vi "SerialReadandWrite.vi"() -> ()   [LabVIEW 2018]
doc: "This example performs writes and reads on a serial port, as directed by the user. You can press the Write and Read buttons, and change the Read Count, while the example is running.\n\nThe parameters set for the serial port must match the parameters of the connected instrument or device. In this example, the Read Count parameter specifies the number of bytes that the serial port reads. If there were more bytes at the port than the specified number, those bytes would not be read. If there were less bytes at the port than the specified number, you would receive a timeout error.\n\nThis example expands upon the flow control options for XON and XOFF, allowing the user to choose those control characters. Also, the user can enable or disable a termination character. Some devices require a termination character in order to identify the end of command strings. Some devices send a termination character to signify the end of data to be read. This example shows how you can end the Read operation once a termination character is detected in the buffer and/or append a termination character at the end of the Write data."
uses:
  Program Files (x86)/National Instruments/LabVIEW 2018/examples/Instrument IO/Serial/support/Serial - Settings.ctl
  <vilib>/Instr/_visa.llb/VISA Configure Serial Port (Instr).vi
panel:
  out "unsigned byte array":u8[](array[numeric])
  in  "VISA resource name":refnum<visa-resource-name>="COM1"
  in  "Serial Settings":T1={"baud rate"=9600, "data bits"=8, "parity"=enum."None", "stop bits"=10, "flow control"=0} {"flow control" items=["None"=0, "XON/XOFF"=1, "RTS/CTS"=2, "DTR/DSR"=4]; "stop bits" items=["1.0"=10, "1.5"=15, "2.0"=20]; "data bits" min=5 max=8 step=1; "baud rate" items=["75"=75, "110"=110, "134"=134, "150"=150, "300"=300, "600"=600, "1200"=1200, "1800"=1800, "2400"=2400, "4800"=4800, "7200"=7200, "9600"=9600, "14400"=14400, "19200"=19200, "28800"=28800, "38400"=38400, "56000"=56000, "57600"=57600, "115200"=115200, "128000"=128000, "230400"=230400]}
  in  "Send Command":bool
  in  "Stop":bool
  in  "Command":string="*IDN?"
  in  "Read Count":u32=1000
  # "Overview: Demonstrates the use of the VISA functions to write commands to and read responses from USB Timestamp Counter (TDC1).\nRequirements: NI-VISA Driver\nInstructions:\n1. Specify the COM port connected to the device.\n2. Run the VI.\n2. Specify a Command and click the Write button.\n3. Read a Response by clicking the Read button.\n4. Click Stop to stop the VI."
  # "0xD is equivalent to a '\\r' character, which is a CR."
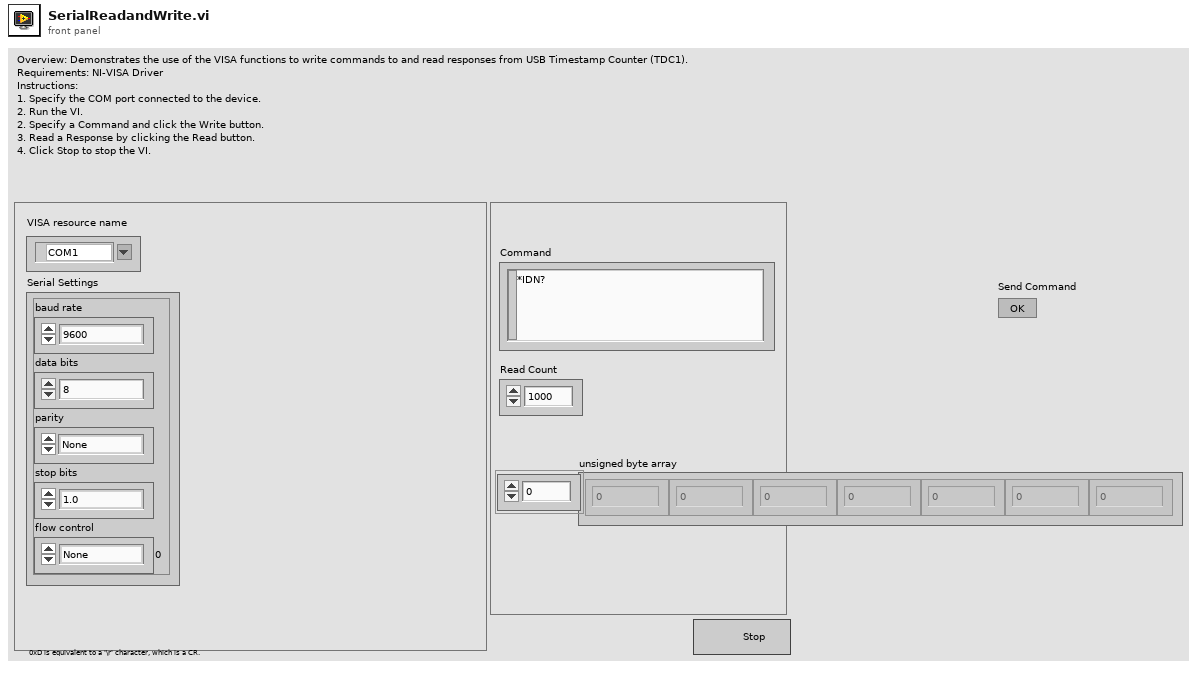
[diagram p1: front panel]
types:
  T1 = typedef "Serial - Settings.ctl" = cluster{"baud rate":u32, "data bits":u16, "parity":enum16{"None", "Odd", "Even", "Mark", "Space"}, "stop bits":u16, "flow control":u16}
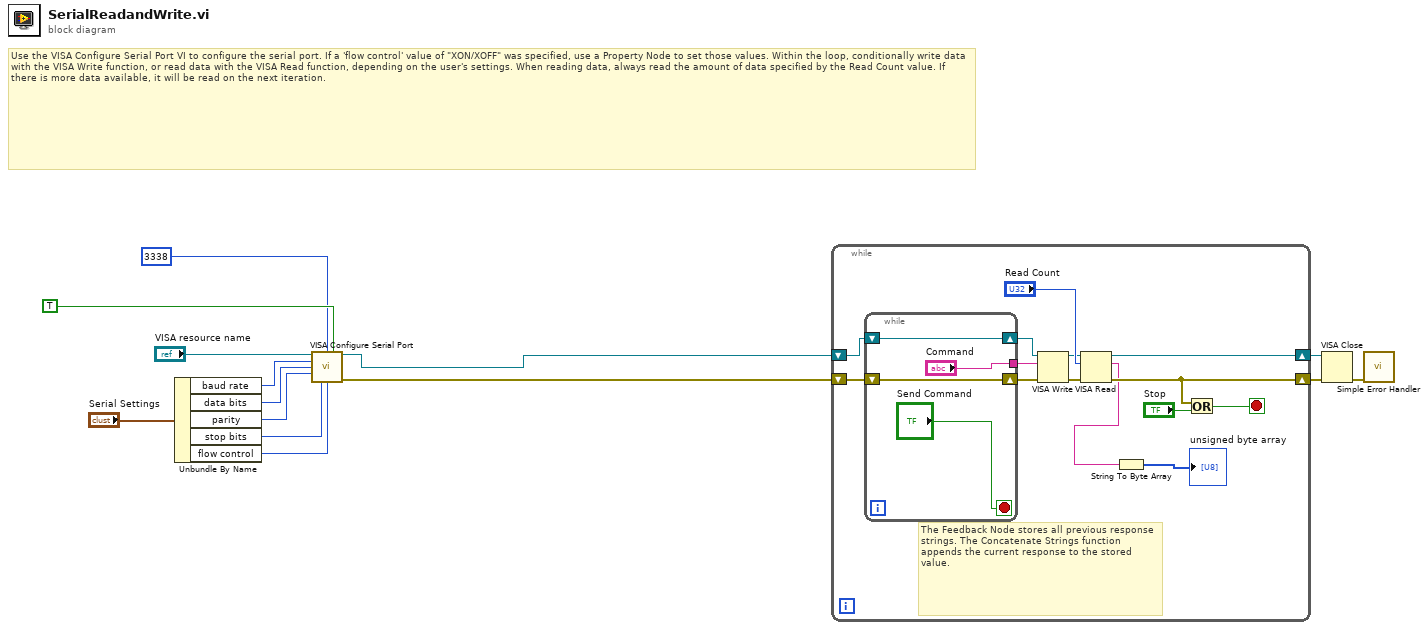
[diagram p0: block diagram]
diagram:
  # "Use the VISA Configure Serial Port VI to configure the serial port. If a 'flow control' value of \"XON/XOFF\" was specified, use a Property Node to set those values. Within the loop, conditionally write data with the VISA Write function, or read data with the VISA Read function, depending on the user's settings. When reading data, always read the amount of data specified by the Read Count value. If there is more data available, it will be read on the next iteration."
  n1 = Unbundle By Name("Serial Settings") -> ("baud rate"=w6:u32, "data bits"=w7:u16, "parity"=w8:enum16{"None", "Odd", "Even", "Mark", "Space"}, "stop bits"=w9:u16, "flow control"=w4:u16)
  n2 = call-poly "VISA Configure Serial Port"("VISA resource name"="VISA resource name", "termination char\n(0xA = '\\n' = LF)"=3338, "Enable Termination\nChar (T)"=TRUE ("End Read on Termination Character?"), "baud rate (9600)"=w6, "data bits (8)"=w7, "parity (0:none)"=w8, "stop bits (10: 1 bit)"=w9, "flow control (0:none)"=w4) -> ("VISA resource name out"=w3:refnum<visa-resource-name>, "error out"=w10:errorcluster)  [unwired: 2 in, 4 out]
  n3 = while {
    shift-right: [w28] -> w13
    shift-left: w10 -> [w26]
    shift-right: [w27] -> w12
    shift-left: w3 -> [w25]
    stop <- w23 stop-if-true
    # "The Feedback Node stores all previous response strings. The Concatenate Strings function appends the current response to the stored value."
    n4 = while {
      shift-right: [w29] -> w20
      shift-left: w26 -> [w29]
      shift-right: [w30] -> w21
      shift-left: w25 -> [w30]
      tunnel: ["Command"] -> w17
      stop <- "Send Command" stop-if-true
    }
    n5 = VISA Write(VISA resource name=w21, write buffer=w17, error in (no error)=w20) -> (VISA resource name out=w18:refnum<visa-resource-name>, error out=w19:errorcluster)  [unwired: 1 out]
    n6 = VISA Read(VISA resource name=w18, byte count="Read Count", error in (no error)=w19) -> (VISA resource name out=w27:refnum<visa-resource-name>, read buffer=w16:string, error out=w28:errorcluster)  [unwired: 1 out]
    n7 = String To Byte Array(string=w16) -> (unsigned byte array=→"unsigned byte array":u8[])
    n8 = Or(x=w28, y="Stop") -> (x .or. y?=w23:bool)
  }
  n9 = VISA Close(VISA resource name=w12, error in (no error)=w13) -> (error out=w14:errorcluster)
  n10 = call <vilib>:"Simple Error Handler.vi"("error in (no error)"=w14) -> ()  [unwired: 1 in, 8 out]
